vi "KE622x -- Get Meas Event Enable Reg State.vi"(0 "VISA Resource In":refnum<visa-resource-name>, 1 "Error Query (T)?":bool=TRUE, 11 "error in (no error)":errorcluster) -> (4 "VISA Resource Out (dupl)":refnum<visa-resource-name>, 8 "KE622x Meas Event Enable Reg":T1, 15 "error out":errorcluster)   [LabVIEW 2009, in "Keithley 622x.lvlib"]
doc: "Returns the bits in the 'Measurement Event Enable' register of the Status Model. Note that only the used (named) bits are returned."
uses:
  <instrlib>/Keithley 622x LV 2009/Utility/Status Registers/Typedefs/KE622x -- Meas Event Enable Reg State.ctl
  <instrlib>/Keithley 622x LV 2009/Keithley 622x.lvlib
panel:
  out "Reg Num (dec)":u16 format="%0d"
  out "Reg Num (binary)":u16 format="%016b"
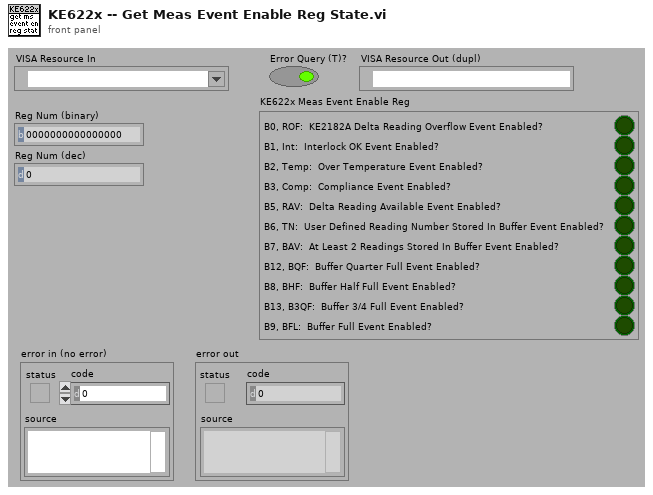
[diagram p1: front panel]
types:
  T1 = typedef "Keithley 622x.lvlib/KE622x -- Meas Event Enable Reg State.ctl" = cluster{"B0, ROF:  KE2182A Delta Reading Overflow Event Enabled?":bool, "B1, Int:  Interlock OK Event Enabled?":bool, "B2, Temp:  Over Temperature Event Enabled?":bool, "B3, Comp:  Compliance Event Enabled?":bool, "B5, RAV:  Delta Reading Available Event Enabled?":bool, "B6, TN:  User Defined Reading Number Stored In Buffer Event Enabled?":bool, "B7, BAV:  At Least 2 Readings Stored In Buffer Event Enabled?":bool, "B12, BQF:  Buffer Quarter Full Event Enabled?":bool, "B8, BHF:  Buffer Half Full Event Enabled?":bool, "B13, B3QF:  Buffer 3/4 Full Event Enabled?":bool, "B9, BFL:  Buffer Full Event Enabled?":bool}
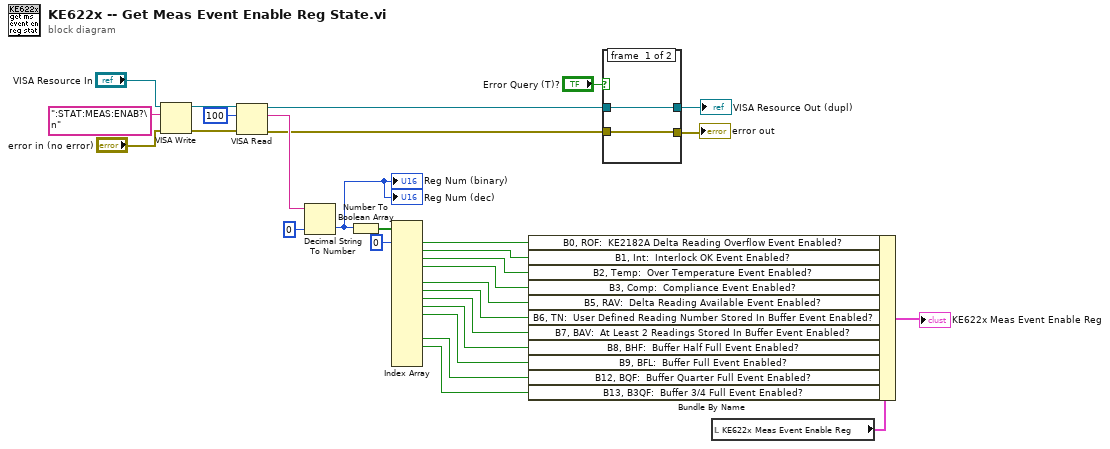
[diagram p0: block diagram]
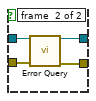
[diagram p2: hidden frame]
diagram:
  n1 = VISA Write(VISA resource name="VISA Resource In", write buffer=":STAT:MEAS:ENAB?\n", error in (no error)="error in (no error)") -> (VISA resource name out=w26:refnum<visa-resource-name>, error out=w25:errorcluster)  [unwired: 1 out]
  n2 = VISA Read(VISA resource name=w26, byte count=u32 100, error in (no error)=w25) -> (VISA resource name out=w14:refnum<visa-resource-name>, read buffer=w23:string, error out=w15:errorcluster)  [unwired: 1 out]
  n3 = Decimal String To Number(string=w23, default (0L)=u16 0 ("default (0 I32)")) -> (number=w19:u16)  [unwired: 2 out]
  "Reg Num (binary)" <- w19
  "Reg Num (dec)" <- w19
  n4 = Number To Boolean Array(number=w19) -> (Boolean array=w21:bool[])
  n5 = Index Array(array=w21, index #1=0 ("index")) -> (element #1=w12:bool, element #2=w11:bool, element #3=w10:bool, element #4=w9:bool, element #6=w7:bool, element #7=w6:bool, element #8=w5:bool, element #9=w4:bool, element #10=w3:bool, element #13=w2:bool, element #14=w1:bool)  [unwired: 15 in, 5 out]
  n6 = case shown="True" "Error Query (T)?" {
    tunnel: w15 -> [w30 w35]
    tunnel: w14 -> [w31 w34]
    tunnel: [w30 w33] -> w16
    tunnel: [w31 w32] -> w17
    frame #0 {
    }
    frame #1 {
      n7 = call <instrlib>:"Error Query.vi"("VISA Resource In"=w34, "error in (no error)"=w35) -> ("VISA Resource Out (dupl)"=w32:refnum<visa-resource-name>, "error out"=w33:errorcluster)  [unwired: 10 in, 2 out]
    }
  }
  "VISA Resource Out (dupl)" <- w17
  "error out" <- w16
  n8 = local read "KE622x Meas Event Enable Reg"() -> (w20:T1)
  n9 = Bundle By Name(cluster=w20, "B0, ROF:  KE2182A Delta Reading Overflow Event Enabled?"=w12, "B1, Int:  Interlock OK Event Enabled?"=w11, "B2, Temp:  Over Temperature Event Enabled?"=w10, "B3, Comp:  Compliance Event Enabled?"=w9, "B5, RAV:  Delta Reading Available Event Enabled?"=w7, "B6, TN:  User Defined Reading Number Stored In Buffer Event Enabled?"=w6, "B7, BAV:  At Least 2 Readings Stored In Buffer Event Enabled?"=w5, "B8, BHF:  Buffer Half Full Event Enabled?"=w4, "B9, BFL:  Buffer Full Event Enabled?"=w3, "B12, BQF:  Buffer Quarter Full Event Enabled?"=w2, "B13, B3QF:  Buffer 3/4 Full Event Enabled?"=w1) -> (→"KE622x Meas Event Enable Reg":T1)
